vi "BME_DG_Errors.vi"(8 "error in (no error)":errorcluster, 10 "source":string="Setting Delays", 11 "error":i32(ring)=503010 items=["Channel refers itself"=503001, "Deadloop"=503002, "Negative Delay"=503003, "Delay Card not found"=503004, "Channel not found"=503005, "Parse Error"=503006, "Not Supported"=503007, "Systen not found"=503008, "To much masters"=503009, "None master in Syterm"=503010, "InterruptError"=503011, "ChnlPeriodeWarning"=503012]) -> (0 "error out":errorcluster)   [LabVIEW 2009, in "POLARIS BME DG.lvlib"]
uses:
  POLARIS BME DG.lvlib
  <vilib>/Utility/error.llb/DialogType.ctl
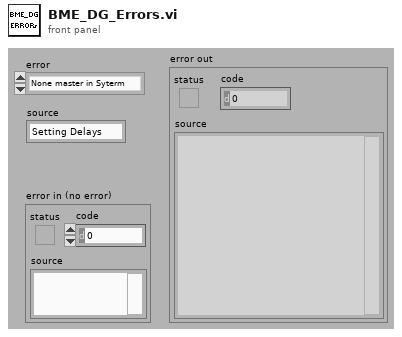
[diagram p1: front panel]
types:
  T1 = typedef "DialogType.ctl" = u16
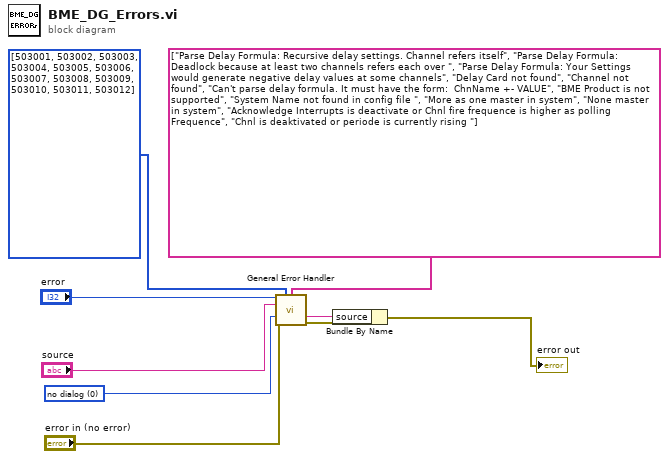
[diagram p0: block diagram]
diagram:
  w5 = T1 0 items=["no dialog", "OK message", "continue or stop message", "OK message + warnings", "continue/stop + warnings"] ("type of dialog (OK msg:1)")
  n1 = call <vilib>:"General Error Handler.vi"("[error code] (0)"="error", "[user-defined codes]"=i32[] [503001, 503002, 503003, 503004, 503005, 503006, 503007, 503008, 503009, 503010, 503011, 503012], "[user-defined descriptions]"=string[] ["Parse Delay Formula: Recursive delay settings. Channel refers itself", "Parse Delay Formula: Deadlock because at least two channels refers each over ", "Parse Delay Formula: Your Settings would generate negative delay values at some channels", "Delay Card not found", "Channel not found", "Can't parse delay formula. It must have the form:  ChnName +- VALUE", "BME Product is not supported", "System Name not found in config file ", "More as one master in system", "None master in system", "Acknowledge Interrupts is deactivate or Chnl fire frequence is higher as polling Frequence", "Chnl is deaktivated or periode is currently rising "], "[error source] (\" \")"="source", "type of dialog (OK msg:1)"=w5, "error in (no error)"="error in (no error)") -> ("message"=w1:string, "error out"=w3:errorcluster)  [unwired: 5 in, 3 out]
  n2 = Bundle By Name(cluster=w3, "source"=w1) -> (→"error out":errorcluster)
